vi "Configure Measurement RRC Filter.vi"(5 "Filter Alpha (0.5)":dbl=0.5 format="%#.6g", 7 "Enable RRC Filter (Disable)":bool, 8 "error in (no error)":errorcluster, 10 "Measurement Method (0: Adjacent Channel Power)":u16(ring) items=["Adjacent Channel Power"=0, "Channel Power"=2, "Multi-Carrier Power"=5, "Spectrum Emissions Mask"=8], 11 "VISA resource name":refnum<visa-resource-name>) -> (0 "error out":errorcluster, 3 "VISA resource name out":refnum<visa-resource-name>)   [LabVIEW 2014, in "Agilent ESA PSA Series.lvlib"]
doc: "Configures RRC Filter. It is only available when either 3GPP W-CDMA or TETRA has been selected as the Radio Standard. If 3GPP W-CDMA is selected, the rolloff value (alpha) for the filter will be initially set to 0.22. T is set to 1/RefBW (default 260 ns). If TETRA is selected, the rolloff will be initially set to 0.35. T is set to 1/RefBW (default 55.56 μs)."
uses:
  Agilent ESA PSA Series.lvlib
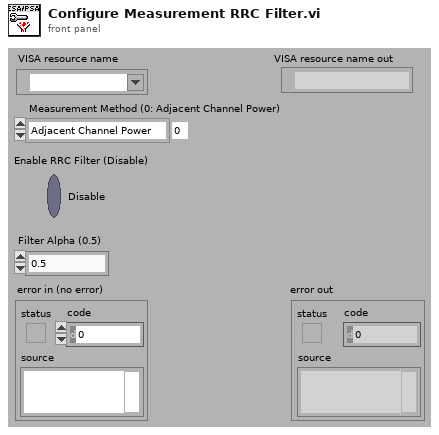
[diagram p1: front panel]
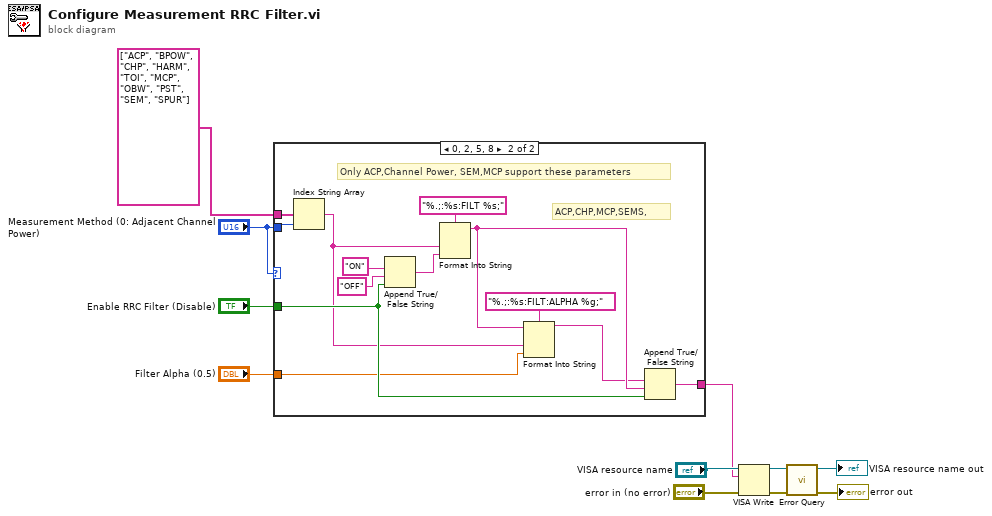
[diagram p0: block diagram]
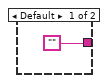
[diagram p2: hidden frame]
diagram:
  n1 = case shown="0, 2, 5, 8" "Measurement Method (0: Adjacent Channel Power)" {
    tunnel: string[] ["ACP", "BPOW", "CHP", "HARM", "TOI", "MCP", "OBW", "PST", "SEM", "SPUR"] -> [_ w25]
    tunnel: "Enable RRC Filter (Disable)" -> [_ w24]
    tunnel: "Filter Alpha (0.5)" -> [_ w23]
    tunnel: "Measurement Method (0: Adjacent Channel Power)" -> [_ w21]
    tunnel: ["" w20] -> w2
    frame Default {
    }
    frame 0, 2, 5, 8 {
      # "Only ACP,Channel Power, SEM,MCP support these parameters"
      # "ACP,CHP,MCP,SEMS,"
      n2 = Index String Array(1:w21, 2:w25) -> (0:w22:string)  [unwired: 1 in]
      n3 = Append True/False String(1:w24, 2:"OFF" ("true string"), 3:"ON" ("true string")) -> (0:w16:string)  [unwired: 1 in]
      n4 = Format Into String(format string="%.;:%s:FILT %s;", w22, w16) -> (resulting string=w14:string)  [unwired: 2 in, 1 out]
      n5 = Format Into String(format string="%.;:%s:FILT:ALPHA %g;", initial string=w14, w22, w23) -> (resulting string=w13:string)  [unwired: 1 in, 1 out]
      n6 = Append True/False String(1:w24, 2:w14, 3:w13) -> (0:w20:string)  [unwired: 1 in]
    }
  }
  n7 = VISA Write(VISA resource name="VISA resource name", write buffer=w2, error in (no error)="error in (no error)") -> (VISA resource name out=w6:refnum<visa-resource-name>, error out=w5:errorcluster)  [unwired: 1 out]
  n8 = call "Error Query.vi"("error in (no error)"=w5, "VISA resource name"=w6) -> ("error out"=→"error out":errorcluster, "VISA resource name out"=→"VISA resource name out":refnum<visa-resource-name>)  [unwired: 6 in, 2 out]
